vi "HasCommand_Query.vi"(0 "System no.":i32=1 min=1 max=4 step=1, 1 "Command":string, 3 "Check HLP?":bool, 4 "HLP? answer":string, 5 "error in":errorcluster) -> (14 "Available GCS commands":string[](array[string]), 15 "Is command available?":bool, 19 "error out":errorcluster)   [LabVIEW 2020]
doc: "Polymorphic VI instance for Is command present in HLP? answer.vi.\nThis VI checks whether the specified command is present in the HLP? answer.\n\nIf Check HLP? is TRUE, HLP?.vi will be called to get HLP? information.\nIf Check HLP? is FALSE, a valid HLP? answer has to be provided in HLP answer."
panel:
  # "Is Command present in HLP answer?.vi\n\nThis VI checks whether the specified command is present in the HLP? answer.\n\nIf \"Check HLP?\" is TRUE, HLP?.vi will be called to get HLP? information.\nIf \"Check HLP?\" is FALSE, a valid HLP? answer has to be provided in \"HLP answer\"."
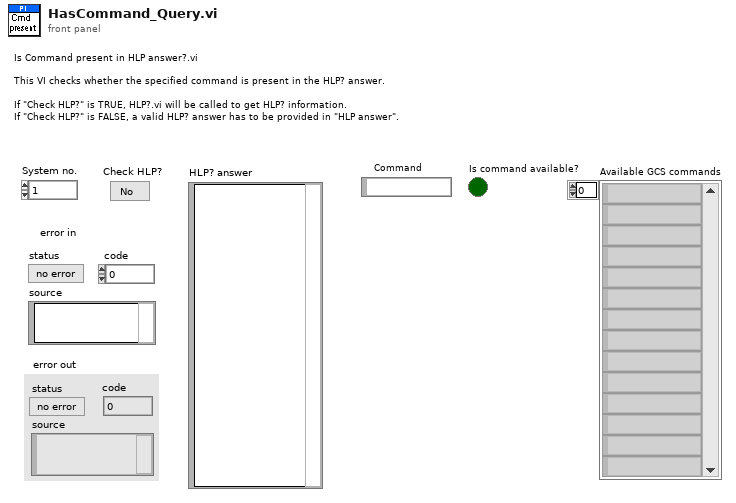
[diagram p1: front panel]
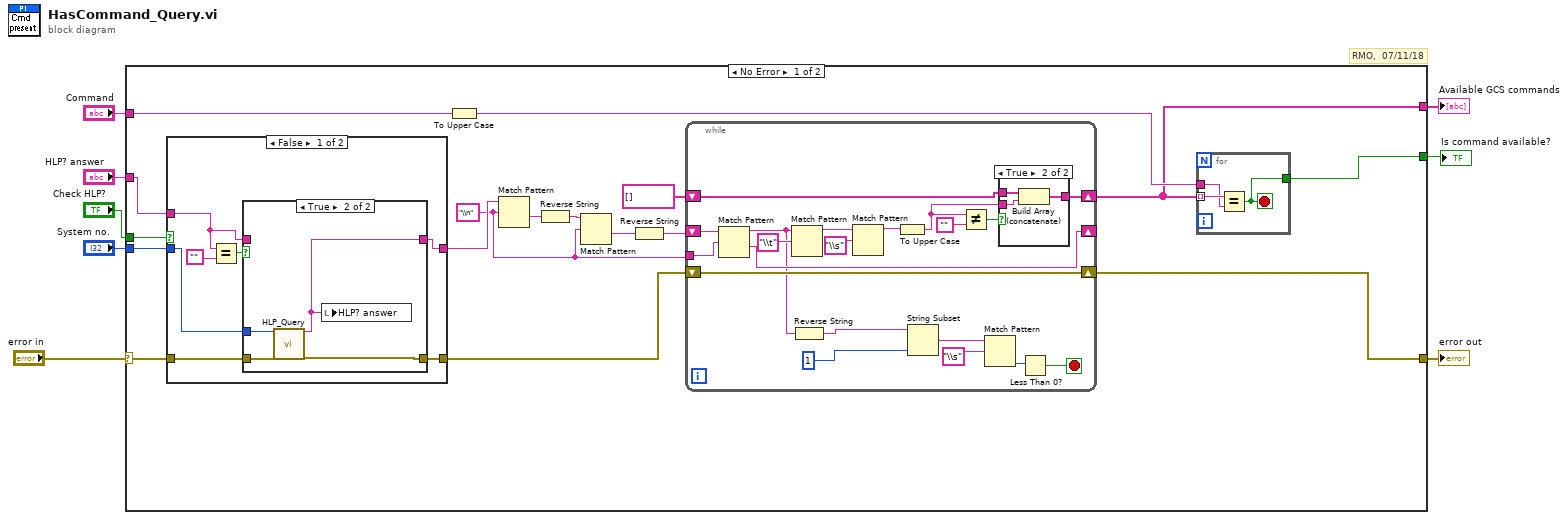
[diagram p0: block diagram]
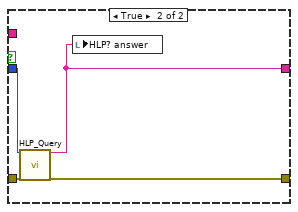
[diagram p3: hidden frame]
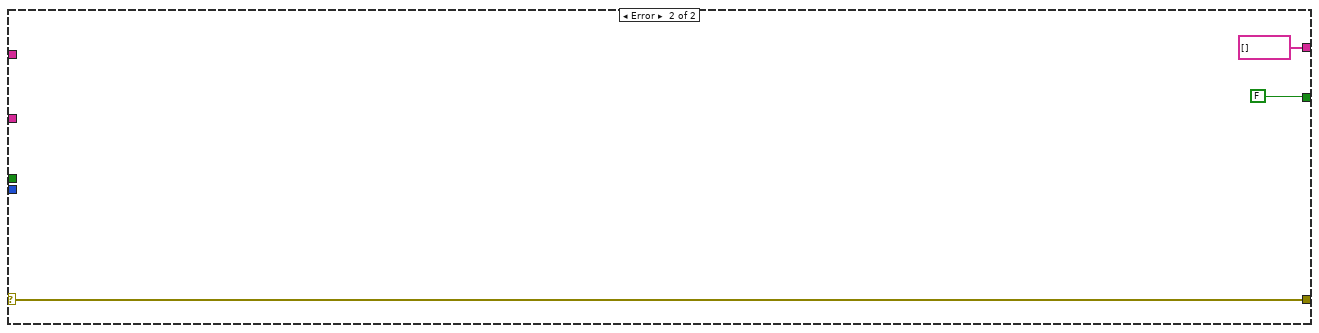
[diagram p5: hidden frame]
diagram:
  # "RMO,  07/11/18"
  n1 = case shown="No Error" "error in" {
    selector: "error in" -> [w9 w70]
    tunnel: [w21 w70] -> w8
    tunnel: "System no." -> [w25 _]
    tunnel: "Command" -> [w13 _]
    tunnel: [w20 string[] []] -> w6
    tunnel: [w10 FALSE] -> w2
    tunnel: "Check HLP?" -> [w12 _]
    tunnel: "HLP? answer" -> [w11 _]
    frame No Error {
      w16 = "\\n" ("regular expression")
      n2 = case shown="False" w12 {
        tunnel: w25 -> [w29 w45]
        tunnel: [w30 w42] -> w19
        tunnel: [w32 w44] -> w14
        tunnel: w9 -> [w33 w43]
        tunnel: w11 -> [w31 _]
        frame False {
          n3 = Equal?(x=w31, y="") -> (x = y?=w34:bool)
          n4 = case shown="True" w34 {
            tunnel: w33 -> [w37 w41]
            tunnel: [w37 w40] -> w32
            tunnel: w31 -> [w36 _]
            tunnel: [w36 w38] -> w30
            tunnel: w29 -> [_ w39]
            frame False {
            }
            frame True {
              n5 = call "HLP_Query.vi"("System no."=w39, "error in"=w41) -> ("Help string"=w38:string, "error out"=w40:errorcluster)  [unwired: 16 out]
              n6 = local write "HLP? answer"(w38) -> ()
            }
          }
        }
        frame True {
          n7 = call "HLP_Query.vi"("System no."=w45, "error in"=w43) -> ("Help string"=w42:string, "error out"=w44:errorcluster)  [unwired: 16 out]
          n8 = local write "HLP? answer"(w42) -> ()
        }
      }
      n9 = To Upper Case(1:w13) -> (0:w22:string)
      n10 = Match Pattern(string=w19, regular expression=w16) -> (after substring=w18:string)  [unwired: 4 out]
      n11 = Reverse String(1:w18) -> (0:w17:string)
      n12 = Match Pattern(string=w17, regular expression=w16) -> (after substring=w15:string)  [unwired: 4 out]
      n13 = Reverse String(1:w15) -> (0:w24:string)
      n14 = while {
        tunnel: w16 -> [w59]
        shift-right: [w55] -> _
        shift-left: w24 -> [w58]
        shift-right: [w63] -> w20
        shift-left: string[] [] -> [w64]
        shift-right: [w57] -> w21
        shift-left: w14 -> [w57]
        stop <- w65 stop-if-true
        n15 = Match Pattern(string=w58, regular expression=w59) -> (before substring=w53:string, after substring=w55:string)  [unwired: 3 out]
        n16 = Match Pattern(string=w53, regular expression="\\t") -> (before substring=w48:string)  [unwired: 4 out]
        n17 = Reverse String(1:w53) -> (0:w52:string)
        n18 = Match Pattern(string=w48, regular expression="\\s") -> (before substring=w46:string)  [unwired: 4 out]
        n19 = To Upper Case(1:w46) -> (0:w62:string)
        n20 = String Subset(string=w52, length (rest)=1) -> (substring=w50:string)  [unwired: 1 out]
        n21 = Not Equal?(x=w62, y="") -> (x != y?=w60:bool)
        n22 = Match Pattern(string=w50, regular expression="\\s") -> (offset past match=w54:i32)  [unwired: 4 out]
        n23 = case shown="True" w60 {
          tunnel: w64 -> [w66 w69]
          tunnel: [w66 w68] -> w63
          tunnel: w62 -> [_ w67]
          frame False {
          }
          frame True {
            n24 = Build Array (concatenate)(w69, w67) -> (w68:string[])
          }
        }
        n25 = Less Than 0?(x=w54) -> (x < 0?=w65:bool)
      }
      n26 = for {
        tunnel: w22 -> [w27]
        tunnel: w20 -> [w28] mode=indexing
        tunnel: [w26] -> w10
        stop <- w26 stop-if-true
        n27 = Equal?(x=w28, y=w27) -> (x = y?=w26:bool)
      }
    }
    frame Error {
    }
  }
  "error out" <- w8
  "Available GCS commands" <- w6
  "Is command available?" <- w2
